vi "vibrate_and_record_async.vi"(3 "SSH password":string, 4 "Transfer and Run Date Folder After Experiment":bool, 5 "SSH user name":string, 6 "Tags":string, 7 "Frames":i32, 8 "frequencies":dbl[](array[numeric]), 9 "PWM duty cycles":dbl[](array[numeric]), 10 "parameters":string[](array[string]), 11 "parameters headers":string[](array[string])) -> ()   [LabVIEW 2014]
uses:
  <vilib>/vision/driver/IMAQdx.llb/IMAQdx Acquisition Mode.ctl
  <vilib>/userdefined/High Color/IMAQdx.ctl
  <vilib>/vision/driver/IMAQdx.llb/IMAQdx Buffer Number Mode.ctl
  <vilib>/Utility/file.llb/Write To Spreadsheet File (DBL).vi
  <vilib>/Utility/file.llb/Write To Spreadsheet File (string).vi
  <vilib>/Utility/file.llb/Read From Spreadsheet File (string).vi
  <vilib>/vision/driver/NI_Vision_Acquisition_Software.lvlib
panel:
  out "ProcessBufferNumber":u32
  out "ProcessFrameRate":dbl
  out "# elements in queue":i32
  out "CameraFrameRate":dbl
  out "Error":string
  out "Save Directory":path
  out "Camera Buffer Number Out":u32
  out "Image":T1(plugin-control)
  in  "stop":bool
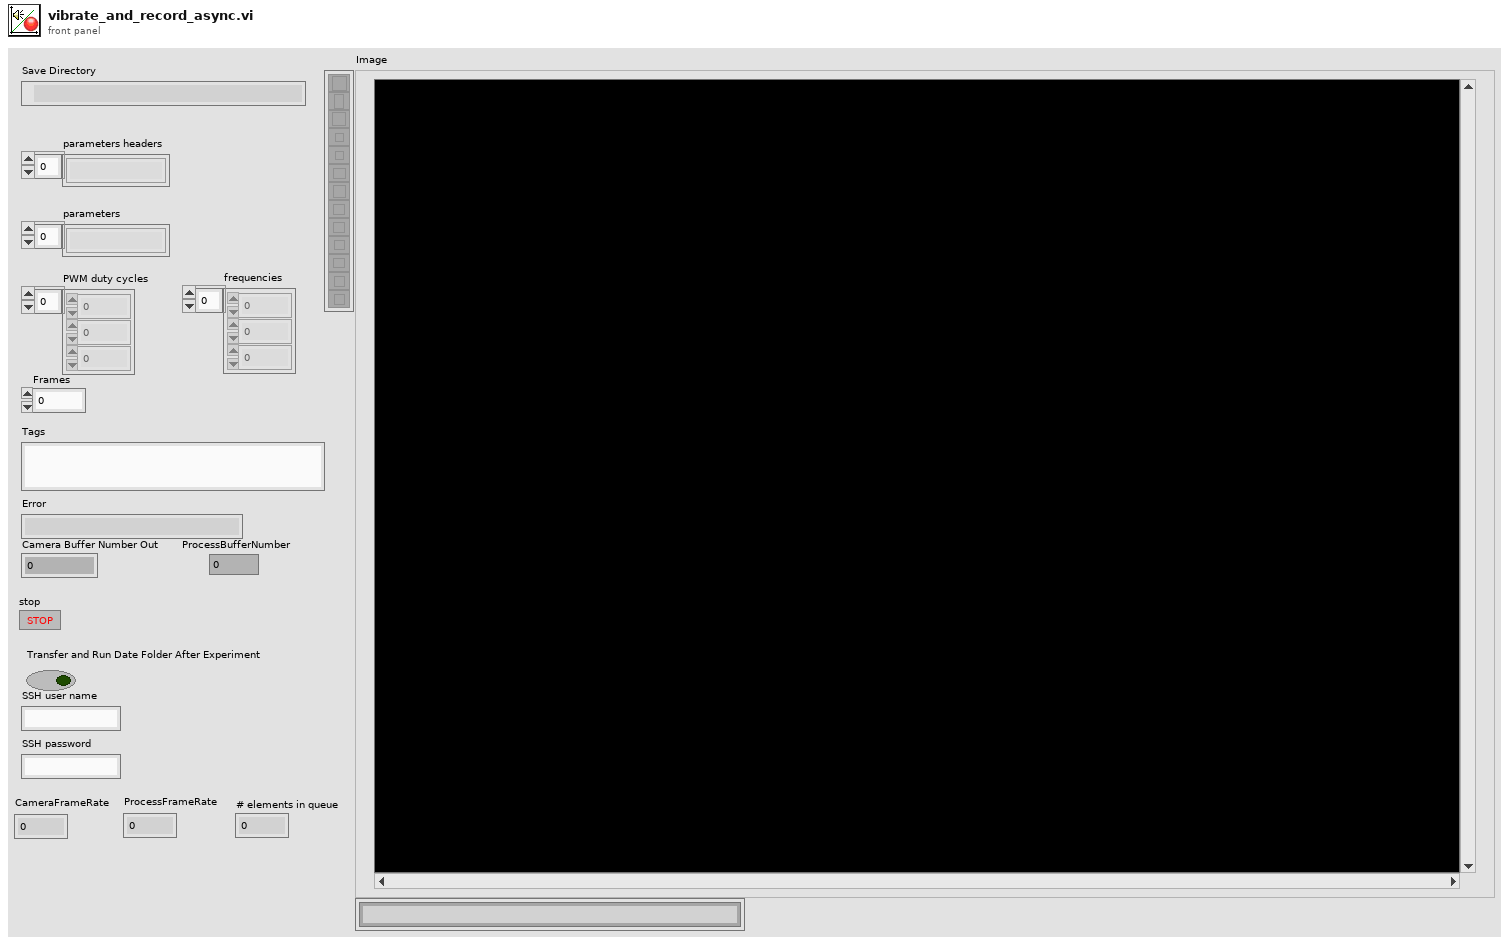
[diagram p1: front panel]
types:
  T1 = typedef "IMAQ Image.ctl" = refnum<image>
  T2 = typedef "IMAQdx.ctl" = refnum<k21>
  T3 = typedef "NI_Vision_Acquisition_Software.lvlib/IMAQdx Buffer Number Mode.ctl" = enum32{"Next", "Last", "Buffer Number"}
  T4 = typedef "Image Type" = u32
  T5 = typedef "NI_Vision_Acquisition_Software.lvlib/IMAQdx Acquisition Mode.ctl" = enum32{"One Shot", "Continuous"}
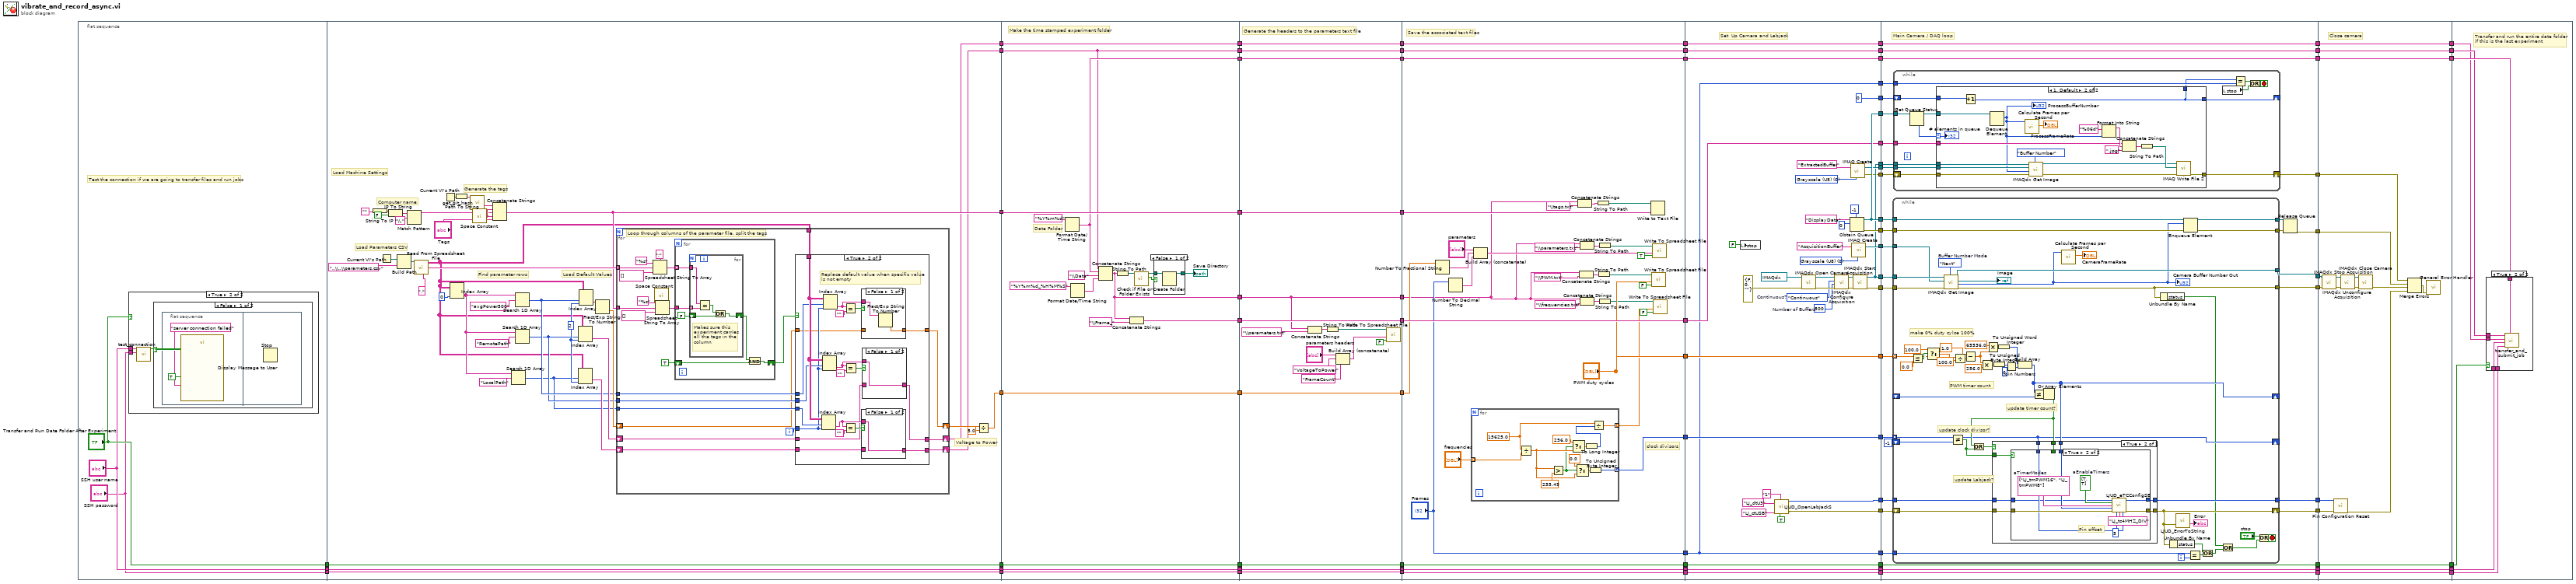
[diagram p0: block diagram]
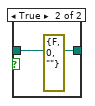
[diagram p8: hidden frame]
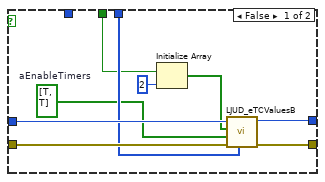
[diagram p11: hidden frame]
diagram:
  n1 = flat-sequence {
    tunnel: ["Transfer and Run Date Folder After Experiment"] -> w44
    tunnel: ["SSH user name"] -> w43
    tunnel: ["SSH password"] -> w42
    tunnel: [w120] -> w74
    tunnel: [w100] -> w73
    tunnel: [w90] -> w64
    tunnel: [w91] -> w63
    tunnel: w44 -> [w111]
    tunnel: w43 -> [w110]
    tunnel: w42 -> [w109]
    tunnel: [w111] -> w35
    tunnel: [w110] -> w28
    tunnel: [w109] -> w27
    tunnel: [w211] -> w58
    tunnel: [w210] -> w56
    tunnel: [w209] -> w54
    tunnel: [w208] -> w52
    tunnel: [w207] -> w50
    tunnel: [w206] -> w48
    tunnel: [w205] -> w46
    tunnel: w63 -> [w205]
    tunnel: w64 -> [w206]
    tunnel: w73 -> [w208]
    tunnel: w74 -> [w209]
    tunnel: [w195] -> w36
    tunnel: w35 -> [w195]
    tunnel: [w194] -> w29
    tunnel: w28 -> [w194]
    tunnel: w27 -> [w193]
    tunnel: [w193] -> w26
    tunnel: w58 -> [w232]
    tunnel: [w232] -> w57
    tunnel: w56 -> [w218]
    tunnel: [w218] -> w55
    tunnel: w54 -> [w231]
    tunnel: [w231] -> w53
    tunnel: w52 -> [w230]
    tunnel: [w230] -> w51
    tunnel: w50 -> [w229]
    tunnel: [w229] -> w49
    tunnel: w48 -> [w228]
    tunnel: [w228] -> w47
    tunnel: w46 -> [w227]
    tunnel: [w227] -> w45
    tunnel: [w217] -> w37
    tunnel: w36 -> [w217]
    tunnel: [w216] -> w30
    tunnel: w29 -> [w216]
    tunnel: w26 -> [w215]
    tunnel: [w215] -> w25
    tunnel: w57 -> [w264]
    tunnel: [w264] -> w79
    tunnel: ["PWM duty cycles"] -> w77
    tunnel: ["Frames"] -> w76
    tunnel: w55 -> [w236]
    tunnel: w53 -> [w247]
    tunnel: w51 -> [w242]
    tunnel: w49 -> [w253]
    tunnel: [w253] -> w69
    tunnel: [w252] -> w65
    tunnel: w47 -> [w252]
    tunnel: [w251] -> w59
    tunnel: w45 -> [w251]
    tunnel: [w245] -> w38
    tunnel: w37 -> [w245]
    tunnel: [w244] -> w31
    tunnel: w30 -> [w244]
    tunnel: w25 -> [w243]
    tunnel: [w243] -> w24
    tunnel: [w233] -> w20
    tunnel: w79 -> [w282]
    tunnel: [w305] -> w81
    tunnel: [w306] -> w80
    tunnel: [w315] -> w78
    tunnel: w77 -> [w315]
    tunnel: w76 -> [w281]
    tunnel: [w281] -> w75
    tunnel: [w313] -> w70
    tunnel: w69 -> [w313]
    tunnel: [w312] -> w66
    tunnel: w65 -> [w312]
    tunnel: [w311] -> w60
    tunnel: w59 -> [w311]
    tunnel: [w310] -> w39
    tunnel: w38 -> [w310]
    tunnel: [w309] -> w32
    tunnel: w31 -> [w309]
    tunnel: w24 -> [w308]
    tunnel: [w308] -> w23
    tunnel: w20 -> [w307]
    tunnel: [w307] -> w19
    tunnel: [w296] -> w16
    tunnel: [w284] -> w15
    tunnel: [w295] -> w14
    tunnel: [w291] -> w11
    tunnel: [w286] -> w10
    tunnel: [w286] -> w9
    tunnel: [w285] -> w8
    tunnel: [w284] -> w7
    tunnel: [w283] -> w6
    tunnel: [w282] -> w5
    tunnel: [w281] -> w4
    tunnel: [0] -> w1
    tunnel: w81 -> [w350]
    tunnel: w80 -> [w349]
    tunnel: w78 -> [w348]
    tunnel: w75 -> [w347]
    tunnel: [w346] -> w71
    tunnel: w70 -> [w346]
    tunnel: [w345] -> w67
    tunnel: w66 -> [w345]
    tunnel: [w344] -> w61
    tunnel: w60 -> [w344]
    tunnel: [w343] -> w40
    tunnel: w39 -> [w343]
    tunnel: [w342] -> w33
    tunnel: w32 -> [w342]
    tunnel: w23 -> [w341]
    tunnel: [w341] -> w22
    tunnel: w19 -> [w338]
    tunnel: [w340] -> w18
    tunnel: [w339] -> w17
    tunnel: w16 -> [w336]
    tunnel: w15 -> [w335]
    tunnel: w14 -> [w334]
    tunnel: [w333] -> w13
    tunnel: [w332] -> w12
    tunnel: w11 -> [w331]
    tunnel: w10 -> [w330]
    tunnel: w9 -> [w327]
    tunnel: w8 -> [w326]
    tunnel: w7 -> [w325]
    tunnel: w6 -> [w324]
    tunnel: w5 -> [w323]
    tunnel: w4 -> [w322]
    tunnel: [w321] -> w3
    tunnel: [w320] -> w2
    tunnel: w1 -> [w319]
    tunnel: [w486] -> w72
    tunnel: w71 -> [w486]
    tunnel: [w485] -> w68
    tunnel: w67 -> [w485]
    tunnel: [w484] -> w62
    tunnel: w61 -> [w484]
    tunnel: [w483] -> w41
    tunnel: w40 -> [w483]
    tunnel: [w482] -> w34
    tunnel: w33 -> [w482]
    tunnel: w22 -> [w481]
    tunnel: [w481] -> w21
    tunnel: w18 -> [w480]
    tunnel: w17 -> [w479]
    tunnel: w13 -> [w474]
    tunnel: w12 -> [w473]
    tunnel: w3 -> [w469]
    tunnel: w2 -> [w468]
    tunnel: w72 -> [w492]
    tunnel: w68 -> [w491]
    tunnel: w62 -> [w490]
    tunnel: w41 -> [w489]
    tunnel: w34 -> [w488]
    tunnel: w21 -> [w487]
    frame #0 {
      # "Test the connection if we are going to transfer files and run jobs"
      n2 = case shown="True" "Transfer and Run Date Folder After Experiment" {
        tunnel: "SSH password" -> [_ w87]
        tunnel: "SSH user name" -> [_ w85]
        frame False {
        }
        frame True {
          n3 = call "test_connection.vi"("Username"=w85, "Password"=w87) -> ("Connection Successful"=w86:bool)  [unwired: 7 in]
          n4 = case shown="False" w86 {
            frame False {
              n5 = flat-sequence {
                frame #0 {
                  n6 = call "Display Message to User"("Enable"=TRUE, "Message"="server connection failed") -> ()  [unwired: 8 in, 2 out]
                }
                frame #1 {
                  n7 = Stop() -> ()  [unwired: 1 in]
                }
              }
            }
            frame True {
            }
          }
        }
      }
    }
    frame #1 {
      w102 = 2
      # "Generate the tags"
      # "Find parameter rows"
      # "Load Default Values"
      # "Voltage to Power"
      # "Load Parameters CSV"
      # "Computer name"
      # "Load Machine Settings"
      n8 = String To IP(1:"") -> (0:w128:u32)
      n9 = Current VI's Path() -> (path=w123:path)
      n10 = IP To String(1:FALSE, 2:w128) -> (0:w125:string)
      n11 = Build Path(base path=w123, name or relative path="..\\..\\parameters.csv") -> (appended path=w113:path)
      n12 = Match Pattern(string=w125, regular expression="\\.") -> (before substring=w103:string)  [unwired: 1 in, 3 out]
      n13 = call-poly <vilib>:"Read From Spreadsheet File.vi"("delimiter (\\t)"=",", "file path (dialog if empty)"=w113) -> ("first row"=w101:string[], "all rows"=w93:string[][])  [unwired: 5 in, 3 out]
      n14 = Current VI's Path() -> (path=w106:path)
      n15 = Index Array(array=w93, index (col)=0) -> (element=w114:string[])  [unwired: 1 in]
      n16 = Path To String(path=w106) -> (string=w105:string)
      n17 = call "get_git_hash.vi"("VI folder"=w105) -> ("github hash"=w108:string)  [unwired: 10 in]
      n18 = call <vilib>:"Space Constant.vi"() -> ("String"=w107:string)
      n19 = Concatenate Strings(w108, w107, w103, w107, "Tags") -> (w100:string)
      n20 = Search 1D Array(1D array=w114, element="LocalPath") -> (index of element=w94:i32)  [unwired: 1 in]
      n21 = Search 1D Array(1D array=w114, element="RemotePath") -> (index of element=w95:i32)  [unwired: 1 in]
      n22 = Search 1D Array(1D array=w114, element="avgPower500") -> (index of element=w96:i32)  [unwired: 1 in]
      n23 = Index Array(array=w93, index (row)=w95, index (col)=w102) -> (element=w98:string)
      n24 = Index Array(array=w93, index (row)=w94, index (col)=w102) -> (element=w97:string)
      n25 = Index Array(array=w93, index (row)=w96, index (col)=w102) -> (element=w116:string)
      n26 = Fract/Exp String To Number(string=w116) -> (number=w99:dbl)  [unwired: 3 in, 1 out]
      n27 = for {
        tunnel: w101 -> [w151] mode=indexing
        tunnel: w100 -> [w143]
        tunnel: w96 -> [w138]
        tunnel: w95 -> [w137]
        tunnel: w94 -> [w136]
        tunnel: w93 -> [w141]
        shift-right: [w133] -> w92
        shift-left: w99 -> [w134]
        shift-right: [w130] -> w91
        shift-left: w98 -> [w131]
        shift-right: [w129] -> w90
        shift-left: w97 -> [w132]
        i -> [w135]
        # "Loop through columns of the parameter file, split the tags"
        n28 = Spreadsheet String To Array(delimiter (Tab)=";", format string="%s", spreadsheet string=w151, array type (2D Dbl)=string[] []) -> (array=w147:string[])
        n29 = call <vilib>:"Space Constant.vi"() -> ("String"=w145:string)
        n30 = Spreadsheet String To Array(delimiter (Tab)=w145, format string="%s", spreadsheet string=w143, array type (2D Dbl)=string[] []) -> (array=w142:string[])
        n31 = for {
          tunnel: w147 -> [w187] mode=indexing
          tunnel: w142 -> [w186]
          shift-right: [w184] -> w139
          shift-left: TRUE -> [w182]
          n32 = for {
            tunnel: w187 -> [w192]
            tunnel: w186 -> [w191] mode=indexing
            shift-right: [w188] -> w183
            shift-left: FALSE -> [w189]
            # "Makes sure this\nexperiment carries\nall the tags in the\ncolumn"
            n33 = Equal?(x=w192, y=w191) -> (x = y?=w190:bool)
            n34 = Or(x=w190, y=w189) -> (x .or. y?=w188:bool)
          }
          n35 = And(x=w183, y=w182) -> (x .and. y?=w184:bool)
        }
        n36 = case shown="True" w139 {
          tunnel: w134 -> [w154 w167]
          tunnel: [w154 w166] -> w133
          tunnel: w138 -> [_ w173]
          tunnel: w137 -> [_ w172]
          tunnel: w136 -> [_ w171]
          tunnel: w135 -> [_ w170]
          tunnel: w141 -> [_ w174]
          tunnel: [w153 w156] -> w130
          tunnel: [w152 w158] -> w129
          tunnel: w132 -> [w152 w157]
          tunnel: w131 -> [w153 w155]
          frame False {
          }
          frame True {
            # "Replace default value when specific value\nis not empty"
            n37 = Index Array(array=w174, index (row)=w171, index (col)=w170) -> (element=w159:string)
            n38 = Index Array(array=w174, index (row)=w172, index (col)=w170) -> (element=w162:string)
            n39 = Index Array(array=w174, index (row)=w173, index (col)=w170) -> (element=w165:string)
            n40 = Equal?(x=w165, y="") -> (x = y?=w168:bool)
            n41 = Equal?(x=w159, y="") -> (x = y?=w160:bool)
            n42 = Equal?(x=w162, y="") -> (x = y?=w163:bool)
            n43 = case shown="False" w168 {
              tunnel: w167 -> [_ w181]
              tunnel: [w180 w181] -> w166
              tunnel: w165 -> [w179 _]
              frame False {
                n44 = Fract/Exp String To Number(string=w179) -> (number=w180:dbl)  [unwired: 3 in, 1 out]
              }
              frame True {
              }
            }
            n45 = case shown="False" w160 {
              tunnel: w159 -> [w175 _]
              tunnel: [w175 w176] -> w158
              tunnel: w157 -> [_ w176]
              frame False {
              }
              frame True {
              }
            }
            n46 = case shown="False" w163 {
              tunnel: w162 -> [w177 _]
              tunnel: [w177 w178] -> w156
              tunnel: w155 -> [_ w178]
              frame False {
              }
              frame True {
              }
            }
          }
        }
      }
      n47 = Divide(x=w92, y=5.0) -> (x/y=w120:dbl)
    }
    frame #2 {
      # "Make the time stamped experiment folder"
      # "Date Folder"
      n48 = Format Date/Time String(time format string (%c)="%Y%m%d") -> (date/time string=w207:string)  [unwired: 2 in]
      n49 = Format Date/Time String(time format string (%c)="%Y%m%d_%H%M%S") -> (date/time string=w199:string)  [unwired: 2 in]
      n50 = Concatenate Strings(w206, w207, "\\Data", w199) -> (w210:string)
      n51 = String To Path(string=w210) -> (path=w198:path)
      n52 = Concatenate Strings(w210, "\\Frame_") -> (w211:string)
      n53 = call <vilib>:"Check if File or Folder Exists.vi"("path"=w198) -> ("file or folder exists?"=w203:bool, "dup path"=w202:path)  [unwired: 8 in, 1 out]
      n54 = case shown="False" w203 {
        tunnel: [w212 w214] -> w197
        tunnel: w202 -> [w213 w214]
        frame False {
          n55 = Create Folder(path (use dialog)=w213) -> (created path=w212:path)  [unwired: 2 in, 2 out]
        }
        frame True {
          (unwired) errorcluster {"status"=FALSE, "code"=0, "source"=""} ("error out")
        }
      }
      "Save Directory" <- w197
    }
    frame #3 {
      # "Generate the headers to the parameters text file"
      n56 = Concatenate Strings(w218, "\\parameters.txt") -> (w226:string)
      n57 = String To Path(string=w226) -> (path=w225:path)
      n58 = Build Array (concatenate)("parameters headers", "VoltageToPower", "FrameCount") -> (w222:string[])
      n59 = call-poly <vilib>:"Write To Spreadsheet File.vi"("append to file? (new file:F)"=FALSE, "1D data"=w222, "file path (dialog if empty)"=w225) -> ()  [unwired: 5 in, 1 out]
    }
    frame #4 {
      # "clock divisors"
      # "Save the associated text files"
      n60 = Number To Fractional String(number=w247) -> (F-format string=w248:string)  [unwired: 3 in]
      n61 = Number To Decimal String(number="Frames") -> (decimal integer string=w249:string)  [unwired: 1 in]
      n62 = for {
        tunnel: [w270] -> w234 mode=indexing
        tunnel: [w269] -> w233 mode=indexing
        tunnel: "frequencies" -> [w268] mode=indexing
        w267 = 15625.0 ("x")
        n63 = Divide(x=w267, y=w268) -> (x/y=w273:dbl)
        n64 = Greater?(x=w273, y=255.49) -> (0:w272:bool)
        n65 = Select(t=256.0, s=w272, f=w273) -> (s? t:f=w275:dbl)
        n66 = Select(t=0.0, s=w272, f=w273) -> (s? t:f=w276:dbl)
        n67 = To Long Integer(number=w275) -> (32bit integer=w271:i32)
        n68 = To Unsigned Byte Integer(number=w276) -> (unsigned 8bit integer=w269:u8)
        n69 = Divide(x=w267, y=w271) -> (x/y=w270:dbl)
      }
      n70 = Build Array (concatenate)("parameters", w248, w249) -> (w257:string[])
      n71 = Concatenate Strings(w236, "\\tags.txt") -> (w255:string)
      n72 = Concatenate Strings(w236, "\\PWM.txt") -> (w266:string)
      n73 = Concatenate Strings(w236, "\\parameters.txt") -> (w261:string)
      n74 = Concatenate Strings(w236, "\\frequencies.txt") -> (w240:string)
      n75 = String To Path(string=w255) -> (path=w254:path)
      n76 = String To Path(string=w266) -> (path=w265:path)
      n77 = String To Path(string=w261) -> (path=w260:path)
      n78 = String To Path(string=w240) -> (path=w239:path)
      n79 = Write to Text File(file (use dialog)=w254, text=w242) -> ()  [unwired: 2 in, 3 out]
      n80 = call-poly <vilib>:"Write To Spreadsheet File.vi"("append to file? (new file:F)"=FALSE, "1D data"="PWM duty cycles", "file path (dialog if empty)"=w265) -> ()  [unwired: 5 in, 1 out]
      n81 = call-poly <vilib>:"Write To Spreadsheet File.vi"("append to file? (new file:F)"=TRUE, "1D data"=w257, "file path (dialog if empty)"=w260) -> ()  [unwired: 5 in, 1 out]
      n82 = call-poly <vilib>:"Write To Spreadsheet File.vi"("append to file? (new file:F)"=FALSE, "1D data"=w234, "file path (dialog if empty)"=w239) -> ()  [unwired: 5 in, 1 out]
    }
    frame #5 {
      w288 = T4 0 items=["Grayscale (U8)", "Grayscale (I16)", "Grayscale (SGL)", "Complex (CSG)", "RGB (U32)", "HSL (U32)", "RGB (U64)"] ("Image Type")
      w301 = T4 0 items=["Grayscale (U8)", "Grayscale (I16)", "Grayscale (SGL)", "Complex (CSG)", "RGB (U32)", "HSL (U32)", "RGB (U64)"] ("Image Type")
      w302 = u32 500  # Number of Buffers
      w298 = IMAQdx_Acquisition_Mode."Continuous"  # Continuous?
      # "Set  Up Camera and Labjack"
      n83 = local write "stop"(FALSE) -> ()
      n84 = call "LJUD_OpenLabJackS.vi"("FirstFound"=TRUE, "Address"="1" ("DeviceType"), "ConnectionType"="LJ_ctUSB", "DeviceType"="LJ_dtU3") -> ("error out"=w306:errorcluster, "Handle"=w305:i32)  [unwired: 5 in, 1 out]
      n85 = call <vilib>:"IMAQdx Open Camera.vi"("error in"=errorcluster {"status"=FALSE, "code"=0, "source"=""}, "Session In"=T2 "cam0") -> ("error out"=w303:errorcluster, "Session Out"=w304:T2)  [unwired: 8 in]
      n86 = call <vilib>:"IMAQdx Configure Acquisition.vi"("error in"=w303, "Number of Buffers"=w302, "Continuous?"=w298, "Session In"=w304) -> ("error out"=w299:errorcluster, "Session Out"=w297:T2)  [unwired: 6 in]
      n87 = Obtain Queue(max queue size (-1, unlimited)=-1, name (unnamed)="DisplayData", element data type=u32 0) -> (queue out=w286:refnum<queue>, error out=w291:errorcluster)  [unwired: 2 in, 1 out]
      n88 = call "IMAQ Create"("Image Name"="ExtractedBuffer", "Image Type"=w288) -> ("New Image"=w285:T1, "error out"=w283:errorcluster)  [unwired: 3 in]
      n89 = call "IMAQ Create"("Image Name"="AcquisitionBuffer", "Image Type"=w301) -> ("New Image"=w295:T1)  [unwired: 3 in, 1 out]
      n90 = call <vilib>:"IMAQdx Start Acquisition.vi"("error in"=w299, "Session In"=w297) -> ("error out"=w296:errorcluster, "Session Out"=w284:T2)  [unwired: 8 in]
    }
    frame #6 {
      # "Main Camera / DAQ loop"
      n91 = while {
        tunnel: w350 -> [w419]
        shift-right: [w412] -> w340
        shift-left: w349 -> [w417]
        tunnel: w348 -> [w404] mode=indexing
        tunnel: w347 -> [w413]
        tunnel: [w418] -> w339
        shift-right: [w411] -> _
        shift-left: _ -> [w423]
        tunnel: w338 -> [w409] mode=indexing
        shift-right: [w409] -> _
        shift-left: -1 -> [w422]
        tunnel: w336 -> [w399]
        tunnel: w335 -> [w398]
        tunnel: w334 -> [w397]
        tunnel: [w396] -> w333
        tunnel: [w395] -> w332
        tunnel: w331 -> [w391]
        tunnel: w330 -> [w390]
        tunnel: [w388] -> w329
        tunnel: [w387] -> w328
        i -> [w416]
        stop <- w438 stop-if-true
        w401 = IMAQdx_Buffer_Number_Mode."Next"  # Buffer Number Mode
        # "make 0% duty cylce 100%"
        # "update timer count?"
        # "update Labjack?"
        # "update clock divisor?"
        # "PWM timer count"
        n92 = Less Or Equal?(x=w404, y=0.0 ("x")) -> (x <= y?=w405:bool)
        n93 = Select(t=100.0 ("y"), s=w405, f=w404) -> (s? t:f=w406:dbl)
        n94 = call <vilib>:"IMAQdx Get Image.vi"("Buffer Number Mode (Next)"=w401, "error in"=w399, "Image In"=w397, "Session In"=w398) -> ("error out"=w396:errorcluster, "Buffer Number Out"=w389:u32, "Image Out"=→"Image":T1, "Session Out"=w395:T2)  [unwired: 4 in]
        "Camera Buffer Number Out" <- w389
        n95 = Not Equal?(x=w409, y=w422) -> (x != y?=w420:bool)
        n96 = Divide(x=w406, y=100.0) -> (x/y=w433:dbl)
        n97 = Subtract(x=1.0, y=w433) -> (x-y=w425:dbl)
        n98 = Multiply(x=w425, y=256.0) -> (x*y=w435:dbl)
        n99 = Multiply(x=65536.0 ("y"), y=w425) -> (x*y=w431:dbl)
        n100 = To Unsigned Byte Integer(number=w435) -> (unsigned 8bit integer=w428:u8)
        n101 = To Unsigned Word Integer(number=w431) -> (unsigned 16bit integer=w430:u16)
        n102 = Join Numbers(hi=w428, lo=u8 0) -> ((hi.lo)=w429:u16)
        n103 = Build Array(w430, w429) -> (w411:u16[])
        n104 = Not Equal?(x=w411, y=w423) -> (x != y?=w424:bool[])
        n105 = Or Array Elements(Boolean array=w424) -> (logical OR=w410:bool)
        n106 = Or(x=w410, y=w420) -> (x .or. y?=w421:bool)
        n107 = case shown="True" w421 {
          tunnel: w420 -> [_ w448]
          tunnel: w419 -> [w440 w447]
          tunnel: [w440 w446] -> w418
          tunnel: w417 -> [w439 w445]
          tunnel: [w439 w444] -> w412
          tunnel: w411 -> [_ w443]
          tunnel: w410 -> [_ w442]
          tunnel: w409 -> [_ w441]
          frame False {
          }
          frame True {
            n108 = case shown="True" w448 {
              tunnel: w447 -> [w454 w458]
              tunnel: [w456 w463] -> w446
              tunnel: w445 -> [w453 w462]
              tunnel: [w457 w461] -> w444
              tunnel: w443 -> [w451 w460]
              tunnel: w442 -> [w450 _]
              tunnel: w441 -> [_ w459]
              frame False {
                w449 = bool[] [TRUE, TRUE]  # aEnableTimers
                n109 = Initialize Array(w450, 2 ("Dimension Size")) -> (w452:bool[])
                n110 = call "LJUD_eTCValuesB.vi"("aTimerValues Write"=w451, "error in"=w453, "aUpdateResetTimers"=w449, "aReadTimers"=w452, "Handle In"=w454) -> ("error out"=w457:errorcluster, "Handle Out"=w456:i32)  [unwired: 3 in, 2 out]
              }
              frame True {
                w465 = bool[] [TRUE, TRUE]  # aEnableTimers
                w467 = string[] ["LJ_tmPWM16", "LJ_tmPWM8"]  # aTimerModes
                # "Pin offset"
                n111 = call "LJUD_eTCConfigSB.vi"("Handle In"=w458, "aEnableTimers"=w465, "aTimerModes"=w467, "aTimerValues"=w460, "error in"=w462, "TCPinOffset"=5, "TimerClockBase"="LJ_tc4MHZ_DIV" ("Timer Clock Base"), "TimerClockDivisor"=w459) -> ("Handle Out"=w463:i32, "error out"=w461:errorcluster)  [unwired: 6 in]
              }
            }
          }
        }
        n112 = call <vilib>:"Calculate Frames per Second.vi"("Buffer Number"=w389) -> ("Processed Frames/s"=→"CameraFrameRate":dbl)  [unwired: 8 in, 2 out]
        n113 = Unbundle By Name(w396) -> ("status"=w402:bool)
        n114 = Unbundle By Name(w412) -> ("status"=w415:bool)
        n115 = call "LJUD_ErrorToString.vi"("error in"=w412) -> ("String"=→"Error":string)  [unwired: 10 in]
        n116 = Enqueue Element(queue=w390, element=w389, error in (no error)=w391) -> (queue out=w387:refnum<queue>, error out=w388:errorcluster)  [unwired: 1 in, 1 out]
        n117 = Equal?(x=w413, y=w416) -> (x = y?=w414:bool)
        n118 = Or(x=w415, y=w414) -> (x .or. y?=w393:bool)
        n119 = Or(x=w402, y=w393) -> (x .or. y?=w394:bool)
        n120 = Or(x="stop", y=w394) -> (x .or. y?=w438:bool)
      }
      n121 = while {
        tunnel: w327 -> [w365]
        tunnel: w326 -> [w362]
        tunnel: w325 -> [w361]
        tunnel: w323 -> [w359]
        shift-right: [w358] -> w320
        shift-left: w324 -> [w360]
        tunnel: w322 -> [w357]
        shift-right: [w352] -> _
        shift-left: w319 -> [w353]
        stop <- w354 stop-if-true
        n122 = Get Queue Status(queue=w365) -> (queue out=w363:refnum<queue>, # elements in queue=w364:i32)  [unwired: 2 in, 6 out]
        n123 = case shown="1, Default" w364 {
          selector: w364 -> [_ w385]
          tunnel: w363 -> [_ w383]
          tunnel: w362 -> [_ w382]
          tunnel: w361 -> [_ w381]
          tunnel: w360 -> [w367 w380]
          tunnel: w359 -> [_ w374]
          tunnel: [w367 w370] -> w358
          tunnel: w353 -> [w366 w369]
          tunnel: [w366 w368] -> w352
          tunnel: [w366 w368] -> w351
          frame 0 {
          }
          frame 1, Default {
            n124 = Increment(x=w369) -> (x+1=w368:i32)
            n125 = Dequeue Element(queue=w383) -> (element=w371:u32)  [unwired: 2 in, 3 out]
            "ProcessBufferNumber" <- w371
            n126 = call <vilib>:"Calculate Frames per Second.vi"("Buffer Number"=w371) -> ("Processed Frames/s"=→"ProcessFrameRate":dbl)  [unwired: 8 in, 2 out]
            n127 = call <vilib>:"IMAQdx Get Image.vi"("Buffer Number Mode (Next)"=IMAQdx_Buffer_Number_Mode."Buffer Number", "error in"=w380, "Buffer Number In"=w371, "Image In"=w382, "Session In"=w381) -> ("error out"=w372:errorcluster, "Image Out"=w373:T1)  [unwired: 3 in, 2 out]
            n128 = Format Into String(format string="%06d" ("string"), w371) -> (resulting string=w376:string)  [unwired: 2 in, 1 out]
            n129 = Concatenate Strings(w374, w376, ".jpg" ("string")) -> (w378:string)
            n130 = String To Path(string=w378) -> (path=w377:path)
            n131 = call-poly "IMAQ Write File 2"("error in (no error)"=w372, "File Path"=w377, "Image"=w373) -> ("error out"=w370:errorcluster)  [unwired: 7 in, 1 out]
            "# elements in queue" <- w385
          }
        }
        n132 = local read "stop"() -> (w355:bool)
        n133 = Equal?(x=w351, y=w357) -> (x = y?=w356:bool)
        n134 = Or(x=w356, y=w355) -> (x .or. y?=w354:bool)
      }
      n135 = Release Queue(queue=w328, error in (no error)=w329) -> (error out=w321:errorcluster)  [unwired: 1 in, 2 out]
    }
    frame #7 {
      # "Close camera"
      n136 = call <vilib>:"IMAQdx Stop Acquisition.vi"("error in"=w474, "Session In"=w473) -> ("error out"=w475:errorcluster, "Session Out"=w476:T2)  [unwired: 8 in]
      n137 = call "Pin Configuration Reset.vi"("error in"=w480, "Handle In"=w479) -> ("error out"=w471:errorcluster)  [unwired: 8 in, 1 out]
      n138 = call <vilib>:"IMAQdx Unconfigure Acquisition.vi"("error in"=w475, "Session In"=w476) -> ("error out"=w478:errorcluster, "Session Out"=w477:T2)  [unwired: 8 in]
      n139 = call <vilib>:"IMAQdx Close Camera.vi"("error in"=w478, "Session In"=w477) -> ("error out"=w470:errorcluster)  [unwired: 9 in]
      n140 = Merge Errors(w468, w469, w470, w471) -> (w472:errorcluster)
      n141 = call <vilib>:"General Error Handler.vi"("error in (no error)"=w472) -> ()  [unwired: 10 in, 5 out]
    }
    frame #8 {
      # "Transfer and run the entire date folder\nif this is the last experiment"
      n142 = case shown="True" w489 {
        tunnel: w492 -> [_ w497]
        tunnel: w491 -> [_ w496]
        tunnel: w490 -> [_ w495]
        tunnel: w488 -> [_ w494]
        tunnel: w487 -> [_ w493]
        frame False {
        }
        frame True {
          n143 = call "transfer_and_submit_job.vi"("Date Folder"=w497, "Password"=w493, "Username"=w494, "Remote Data Directory"=w495, "Local Data Directory"=w496) -> ()  [unwired: 7 in]
        }
      }
    }
  }
